vi "LINC Generate GUID.vi"() -> (0 "GUID":string)   [LabVIEW 2018, in "STEPkgDriver_LINC.lvlib"]
uses:
  STEPkgDriver_LINC.lvlib
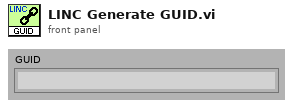
[diagram p1: front panel]
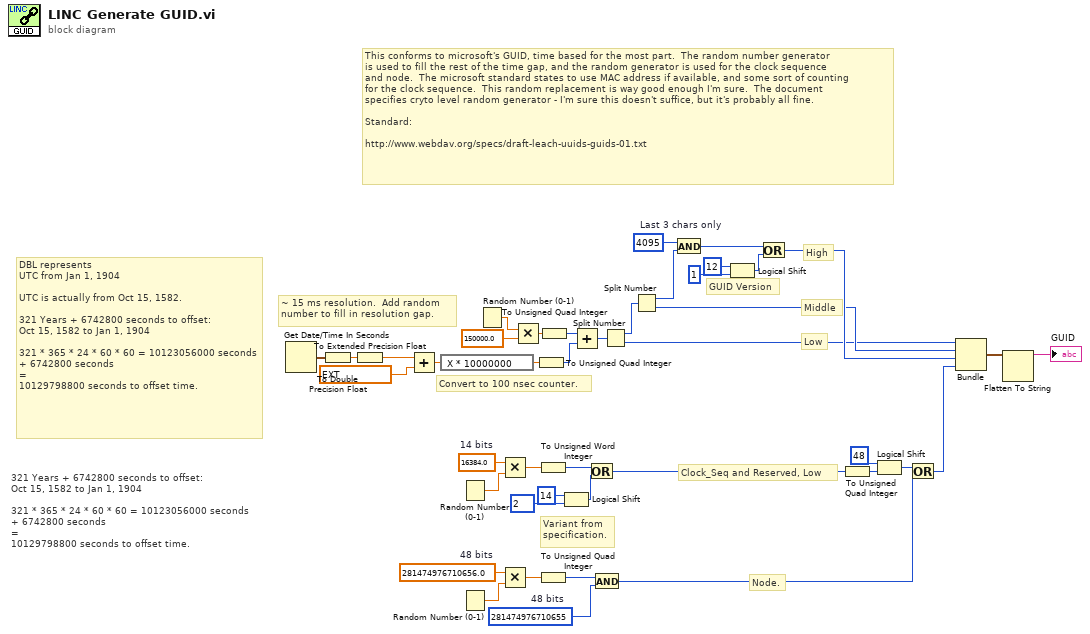
[diagram p0: block diagram]
diagram:
  w38 = u64 281474976710655  # 48 bits
  w36 = 281474976710656.0  # 48 bits
  w27 = 16384.0  # 14 bits
  w16 = u16 4095  # Last 3 chars only
  # "This conforms to microsoft's GUID, time based for the most part.  The random number generator\nis used to fill the rest of the time gap, and the random generator is used for the clock sequence\nand node.  The microsoft standard states to use MAC address if available, and some sort of counting\nfor the clock sequence.  This random replacement is way good enough I'm sure.  The document\nspecifies cryto level random generator - I'm sure this doesn't suffice, but it's probably all fine.\n\nStandard:\n\nhttp://www.webdav.org/specs/draft-leach-uuids-guids-01.txt"
  # "Node."
  # "Clock_Seq and Reserved, Low"
  # "Variant from\nspecification."
  # "Low"
  # "Middle"
  # "High"
  # "GUID Version"
  # "~ 15 ms resolution.  Add random\nnumber to fill in resolution gap."
  # "Convert to 100 nsec counter."
  # "321 Years + 6742800 seconds to offset:\nOct 15, 1582 to Jan 1, 1904\n\n321 * 365 * 24 * 60 * 60 = 10123056000 seconds\n+ 6742800 seconds\n=\n10129798800 seconds to offset time."
  # "DBL represents\nUTC from Jan 1, 1904\n\nUTC is actually from Oct 15, 1582.\n\n321 Years + 6742800 seconds to offset:\nOct 15, 1582 to Jan 1, 1904\n\n321 * 365 * 24 * 60 * 60 = 10123056000 seconds\n+ 6742800 seconds\n=\n10129798800 seconds to offset time."
  n1 = Get Date/Time In Seconds() -> (seconds since 1Jan1904=w8:timestamp)
  n2 = To Double Precision Float(number=w8) -> (double precision float=w9:dbl)
  n3 = To Extended Precision Float(1:w9) -> (0:w10:ext)
  n4 = Add(x=w10, y=ext 10129798800.0) -> (x+y=w12:ext)
  n5 = expression code="X * 10000000"(w12) -> (w13:ext)
  n6 = Random Number (0-1)() -> (number: 0 to 1=w28:dbl)
  n7 = Random Number (0-1)() -> (number: 0 to 1=w35:dbl)
  n8 = Random Number (0-1)() -> (number: 0 to 1=w21:dbl)
  n9 = Multiply(x=w27, y=w28) -> (x*y=w29:dbl)
  n10 = Multiply(x=w36, y=w35) -> (x*y=w34:dbl)
  n11 = Multiply(x=w21, y=150000.0 ("Count32L")) -> (x*y=w23:dbl)
  n12 = To Unsigned Quad Integer(1:w13) -> (0:w25:u64)
  n13 = To Unsigned Word Integer(number=w29) -> (unsigned 16bit integer=w30:u16)
  n14 = To Unsigned Quad Integer(1:w34) -> (0:w37:u64)
  n15 = To Unsigned Quad Integer(1:w23) -> (0:w24:u64)
  n16 = Logical Shift(y=u16 14, x=u16 2) -> (x << y=w33:u16)
  n17 = Add(x=w24, y=w25) -> (x+y=w26:u64)
  n18 = Or(x=w30, y=w33) -> (x .or. y?=w3:u16)
  n19 = And(x=w37, y=w38) -> (x .and. y?=w4:u64)
  n20 = Split Number(x=w26) -> (hi(x)=w14:u32, lo(x)=w39:u32)
  n21 = Split Number(x=w14) -> (hi(x)=w15:u16, lo(x)=w40:u16)
  n22 = And(x=w16, y=w15) -> (x .and. y?=w20:u16)
  n23 = Logical Shift(y=u16 12, x=u16 1) -> (x << y=w17:u16)
  n24 = Or(x=w20, y=w17) -> (x .or. y?=w41:u16)
  n25 = To Unsigned Quad Integer(1:w3) -> (0:w7:u64)
  n26 = Logical Shift(y=i8 48, x=w7) -> (x << y=w5:u64)
  n27 = Or(x=w5, y=w4) -> (x .or. y?=w2:u64)
  n28 = Bundle(w39, w40, w41, w2) -> (w42:cluster{u32, u16, u16, u64})  [unwired: 1 in]
  n29 = Flatten To String(anything=w42) -> (data string=→"GUID":string)  [unwired: 3 in, 2 out]
